vi "Convert Buffer to T&H.vi"(11 "buffer":u8[](array[numeric])) -> (2 "Humidity":dbl, 3 "Temperature":dbl)   [LabVIEW 2019, in "TEMPerHUM.lvlib"]
uses:
  TEMPerHUM.lvlib
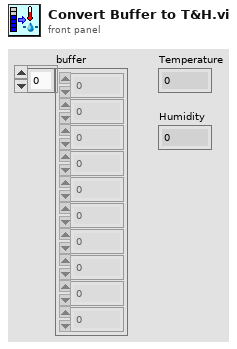
[diagram p1: front panel]
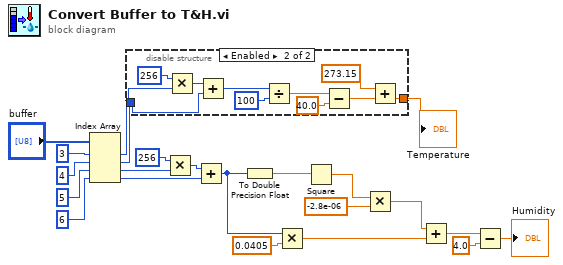
[diagram p0: block diagram]
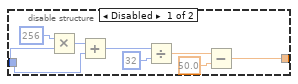
[diagram p2: hidden frame]
diagram:
  n1 = Index Array(array="buffer", index #1=3 ("index"), index #2=4 ("index"), index #3=5 ("index"), index #4=6 ("index")) -> (element #1=w18:u8, element #2=w17:u8, element #3=w13:u8, element #4=w12:u8)
  n2 = disable-structure shown="Enabled" {
    disable-tunnel: w18 -> [w27 w37]
    disable-tunnel: w17 -> [w24 w34]
    disable-tunnel: [w23 w33] -> w1
    frame Disabled {
      n3 = Multiply(x=i16 256, y=w27) -> (x*y=w25:i16)
      n4 = Add(x=w25, y=w24) -> (x+y=w26:i16)
      n5 = Divide(x=w26, y=i16 32) -> (x/y=w29:dbl)
      n6 = Subtract(x=w29, y=50.0) -> (x-y=w23:dbl)
    }
    frame Enabled {
      n7 = Multiply(x=i16 256, y=w37) -> (x*y=w35:i16)
      n8 = Add(x=w35, y=w34) -> (x+y=w36:i16)
      n9 = Divide(x=w36, y=i16 100) -> (x/y=w39:dbl)
      n10 = Subtract(x=w39, y=40.0) -> (x-y=w42:dbl)
      n11 = Add(x=273.15, y=w42) -> (x+y=w33:dbl)
    }
  }
  "Temperature" <- w1
  n12 = Multiply(x=i16 256, y=w13) -> (x*y=w11:i16)
  n13 = Add(x=w11, y=w12) -> (x+y=w4:i16)
  n14 = To Double Precision Float(number=w4) -> (double precision float=w3:dbl)
  n15 = Multiply(x=w4, y=0.0405) -> (x*y=w8:dbl)
  n16 = Square(x=w3) -> (x^2=w5:dbl)
  n17 = Multiply(x=w5, y=-2.8e-06) -> (x*y=w2:dbl)
  n18 = Add(x=w2, y=w8) -> (x+y=w7:dbl)
  n19 = Subtract(x=w7, y=4.0) -> (x-y=→"Humidity":dbl)
